vi "main.vi"() -> ()   [LabVIEW 2013]
panel:
  out "Numeric":dbl
  out "main loop":i32
  in  "stop":bool
  in  "OK Button":bool
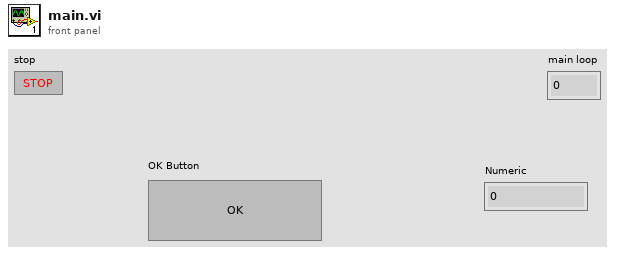
[diagram p1: front panel]
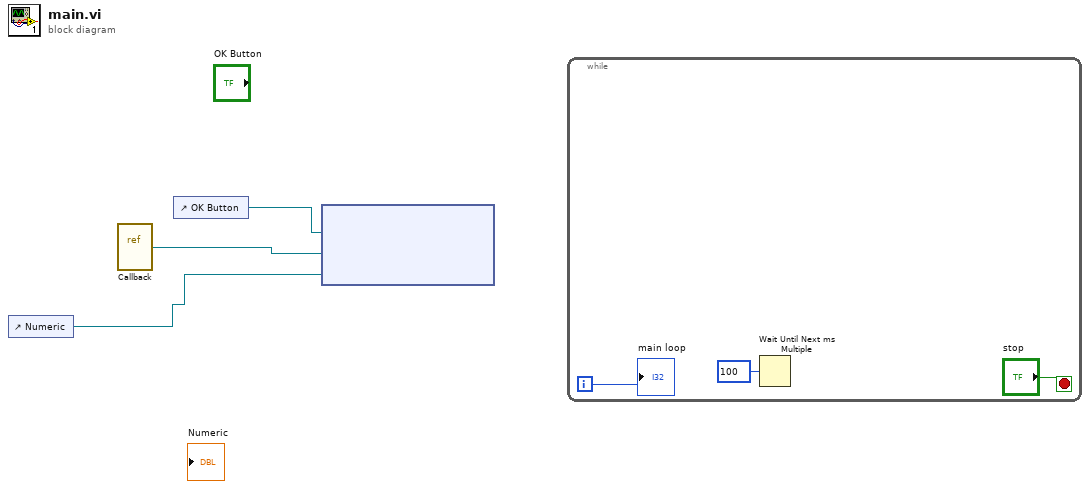
[diagram p0: block diagram]
diagram:
  n1 = control-ref of="Numeric"() -> (w2:refnum<vi>)
  n2 = vi-ref "Callback.vi"() -> ("vi reference"=w1:refnum<vi>)
  n3 = control-ref of="OK Button"() -> (w3:refnum<vi>)
  n4 = node(w3, w1, w2) -> ()  [unwired: 2 in, 2 out]
  n5 = while {
    i -> [w4]
    stop <- "stop" stop-if-true
    n6 = Wait Until Next ms Multiple(millisecond multiple=u32 100) -> ()  [unwired: 1 out]
    "main loop" <- w4
  }
